vi "raw_to_calibrated_configuration-array.vi"(5 "tag_names []":string[](array[string]), 7 "configuration":T1[](array[typedef]), 8 "error in (no error)":errorcluster, 11 "value in":dbl[](array[numeric])) -> (0 "error out":errorcluster, 3 "value out":dbl[](array[numeric]))   [LabVIEW 2015, in "lv-calibration.lvlib"]
uses:
  lv-calibration.lvlib
  <userlib>/antonio-alexander/lv-calibration/public/_controls/configuration.ctl
  _controls/type.ctl
  <userlib>/antonio-alexander/lv-calibration/public/_controls/point.ctl
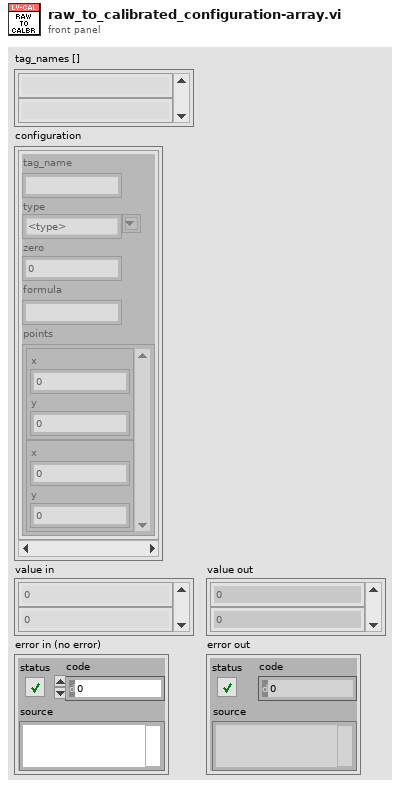
[diagram p1: front panel]
types:
  T1 = typedef "configuration.ctl" = cluster{"tag_name":string, "type":T2, "zero":dbl, "formula":string, "points":T3[]}
  T2 = typedef "lv-calibration.lvlib/type.ctl" = string
  T3 = typedef "point.ctl" = cluster{"x":dbl, "y":dbl}
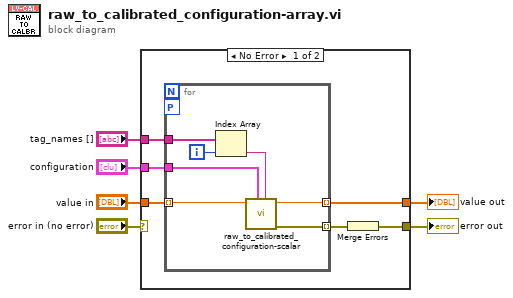
[diagram p0: block diagram]
diagram:
  n1 = case shown="No Error" "error in (no error)" {
    selector: "error in (no error)" -> [_ w20]
    tunnel: "value in" -> [w11 _]
    tunnel: [w7 w20] -> w5
    tunnel: "configuration" -> [w9 _]
    tunnel: "tag_names []" -> [w8 _]
    tunnel: [w10 _] -> w1
    frame No Error {
      n2 = for {
        tunnel: w11 -> [w18] mode=indexing
        tunnel: [w17] -> w10 mode=indexing
        tunnel: w9 -> [w13]
        tunnel: w8 -> [w16]
        tunnel: [w19] -> w12 mode=indexing
        workers-P: _ -> [_]
        i -> [w14]
        n3 = Index Array(array=w16, index=w14) -> (element=w15:string)
        n4 = call "raw_to_calibrated_configuration-scalar.vi"("tag_name"=w15, "configuration"=w13, "value in"=w18) -> ("error out"=w19:errorcluster, "value out"=w17:dbl)  [unwired: 7 in]
      }
      n5 = Merge Errors(w12) -> (w7:errorcluster)
    }
    frame Error {
    }
  }
  "error out" <- w5
  "value out" <- w1
